vi "Read CurrentGame.vi"(8 "error in (no error)":errorcluster, 11 "Engine in":refnum<class "Engine.lvclass">) -> (0 "error out":errorcluster, 2 "RT_Game.lvlib:Game.lvclass":refnum<class "Game.lvclass">, 3 "Engine out":refnum<class "Engine.lvclass">)   [LabVIEW 2019, in "RT_Game.lvlib" / "Engine.lvclass"]
uses:
  Engine.lvclass
  Game/Game.lvclass
  Engine.lvclass/Engine.ctl
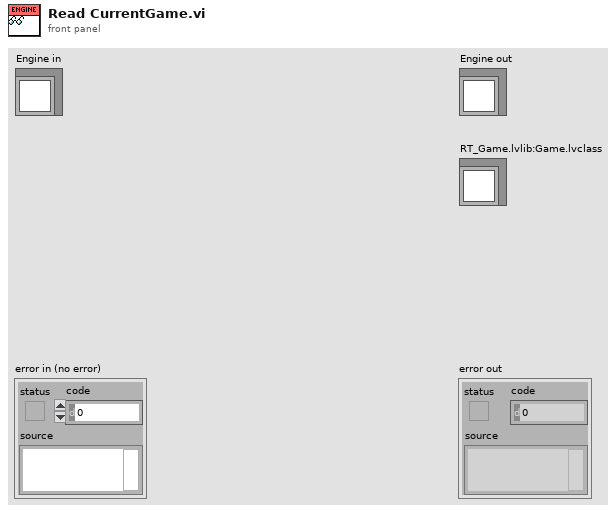
[diagram p1: front panel]
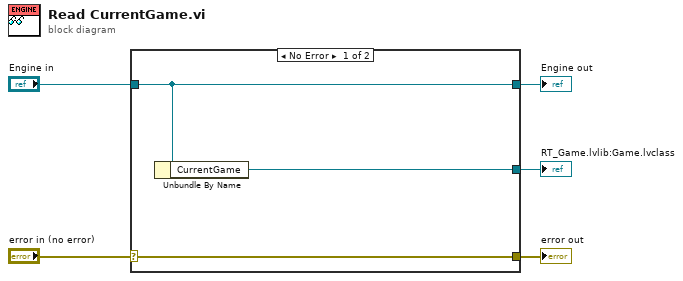
[diagram p0: block diagram]
diagram:
  n1 = case shown="No Error" "error in (no error)" {
    selector: "error in (no error)" -> [w8 w9]
    tunnel: [w8 w9] -> w4
    tunnel: [w7 w10] -> w2
    tunnel: "Engine in" -> [w7 w10]
    tunnel: [w6 _] -> w1
    frame No Error {
      n2 = Unbundle By Name(w7) -> ("CurrentGame"=w6:refnum<class "Game.lvclass">)
    }
    frame Error {
    }
  }
  "error out" <- w4
  "Engine out" <- w2
  "RT_Game.lvlib:Game.lvclass" <- w1
